vi "Main.vi"() -> ()   [LabVIEW 2018]
uses:
  Controls/1D_2D.ctl
  Controls/Rows_Columns.ctl
  Controls/Lengths_Rows_Columns.ctl
  Controls/E_S.ctl
panel:
  in  "Tab Control":T1(tab)
  in  "Choose Array Size":T2
  in  "Array Size 1D":i8[](array[numeric])=[0, 1, 2, 3]
  in  "Array Size 2D":i8[][](array[numeric])=[[0, 4, 8], [1, 5, 9], [2, 6, 10], [3, 7, 11]]
  out "Size 1D":i32
  out "Size 2D":T3
  in  "Index 1D":i32
  in  "Indexs":T3={"Rows"=-1, "Columns"=-1} {"Columns" min=-1; "Rows" min=-1}
  in  "Index Array 1D":i8[](array[numeric])=[1, 3, 4, -2, 0, 10]
  in  "Index Array 2D":i8[][](array[numeric])=[[0, 4, -3], [1, 5, -4], [2, -1, -5], [3, -2, 100]]
  out "Index Value":i8
  out "Index SubArray":i8[](array[numeric])
  in  "Choose Index Array":T2
  in  "E or S Index Array":T4
  in  "Choose RAS":T2
  in  "Element RAS":i8=-10
  in  "E or S RAS":T4
  in  "Subarray RAS":i8[](array[numeric])=[-5, -8]
  in  "Index RAS":i32
  in  "RAS1D":i8[](array[numeric])=[100, -1, -2, 9, 10]
  in  "RAS2D":i8[][](array[numeric])=[[0, 4, 7], [0, 5, 8], [3, 6, 9]]
  in  "Indexs RAS":T3={"Rows"=-1, "Columns"=-1} {"Columns" min=-1; "Rows" min=-1}
  out "New Array RAS1D":i8[](array[numeric])
  out "New Array RAS2D":i8[][](array[numeric])
  in  "Choose IIA":T2
  in  "E or S IIA":T4
  in  "Index IIA":i32
  in  "Element IIA":i8
  in  "SubArray IIA":i8[](array[numeric])=[-1, -2]
  in  "Insert Into Array 1D":i8[](array[numeric])=[1, 2, 3, 4]
  out "Array 1D IIA":i8[](array[numeric])=[1, 2, 3, 4]
  in  "SubArray IIA 2D":i8[][](array[numeric])=[[-10, -12], [-11, -13]]
  in  "Indexs IIA":T3={"Rows"=-1, "Columns"=-1}
  in  "Insert Into Array 2D":i8[][](array[numeric])=[[0, 3, 6], [1, 4, 7], [2, 5, 8]]
  out "Array 2D IIA":i8[][](array[numeric])
  in  "Choose delete from array":T2
  in  "Length":i32
  in  "Index Delete":i32
  in  "Delete from Array 1D":i8[](array[numeric])=[0, 1, 2, 3, 4]
  in  "Indexs DFA":T3={"Rows"=-1, "Columns"=-1} {"Columns" min=-1; "Rows" min=-1}
  out "New Array 1D":i8[](array[numeric])
  out "Deleted Portion 1D":i8[](array[numeric])
  in  "Delete from Array 2D":i8[][](array[numeric])=[[-5, -1, 3], [-4, 0, 4], [-3, 1, 5], [-2, 2, 6]]
  out "New Array 2D":i8[][](array[numeric])
  out "Deleted Portion 2D":i8[][](array[numeric])
  in  "Choose Initialize Array":T2
  in  "Value":i8
  in  "Dimension 1D Array":i32
  in  "Dimensions for 2D":T3
  out "Initialized Array 1D":i8[](array[numeric])
  out "Initialized Array 2D":i8[][](array[numeric])
  in  "Choose Subset Array":T2
  in  "Index Subset":i32
  in  "Subset Array 1D":i8[](array[numeric])=[0, 1, 2, 3, 4]
  out "SubArray 1D":i8[](array[numeric])
  in  "Length Subset":i32
  in  "Indexs SA":T3={"Rows"=-1, "Columns"=-1} {"Columns" min=-1; "Rows" min=-1}
  in  "Lengths R&C":T5
  in  "Subset Array 2D":i8[][](array[numeric])=[[-5, -1, 3], [-4, 0, 4], [-3, 1, 5], [-2, 2, 6]]
  out "SubArray 2D":i8[][](array[numeric])
  in  "Max & Min Array 1D":i8[](array[numeric])=[1, -1, 2, 100, 10]
  in  "Max & Min Array 2D":i8[][](array[numeric])=[[-3, 55, 41], [6, -1, 14], [-3, 2, -70], [-100, 1, 7]]
  in  "Choose Max & Min Array":T2
  out "Max. Value":i8
  out "Indexs Min.":T3
  out "Index Max.":i32
  out "Indexs Max.":T3
  out "Min. Value":i8
  out "Index Min.":i32
  in  "Sort Array":i8[](array[numeric])=[3, 9, 8, 11, 100, 14]
  out "Sorted Array":i8[](array[numeric])=[3, -7, 8, -3, 100, 14]
  # "Usarán el Tab Control\npara ordenar los controles\ne indicadores necesarios para\ncada sección de la tarea"
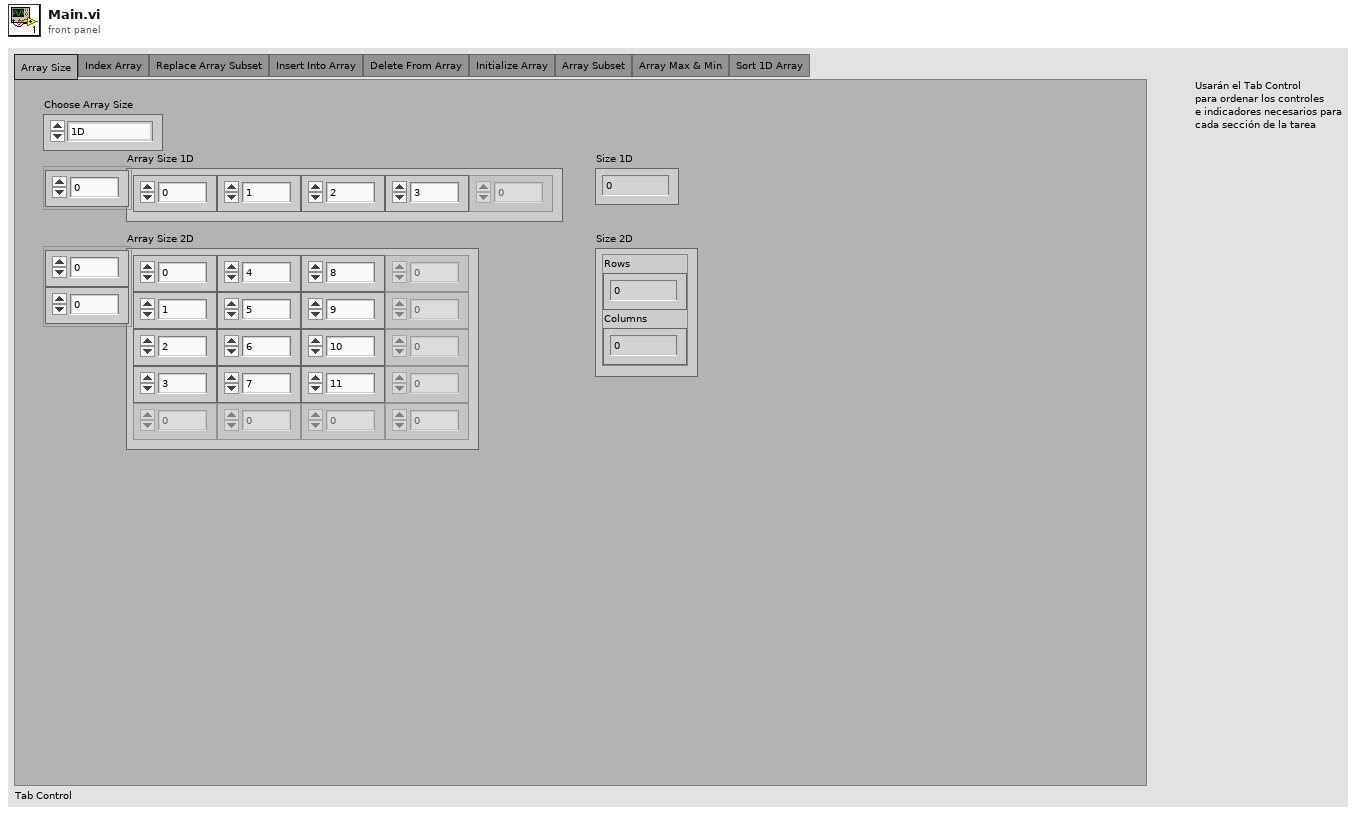
[diagram p1: front panel]
types:
  T1 = enum32{"Array Size", "Index Array", "Replace Array Subset", "Insert Into Array", "Delete From Array", "Initialize Array", "Array Subset", "Array Max & Min", "Sort 1D Array"}
  T2 = typedef "1D_2D.ctl" = enum16{"1D", "2D"}
  T3 = typedef "Rows_Columns.ctl" = cluster{"Rows":i32, "Columns":i32}
  T4 = typedef "E_S.ctl" = enum16{"Element", "SubArray"}
  T5 = typedef "Lengths_Rows_Columns.ctl" = cluster{"Length Rows":i32, "Length Columns":i32}
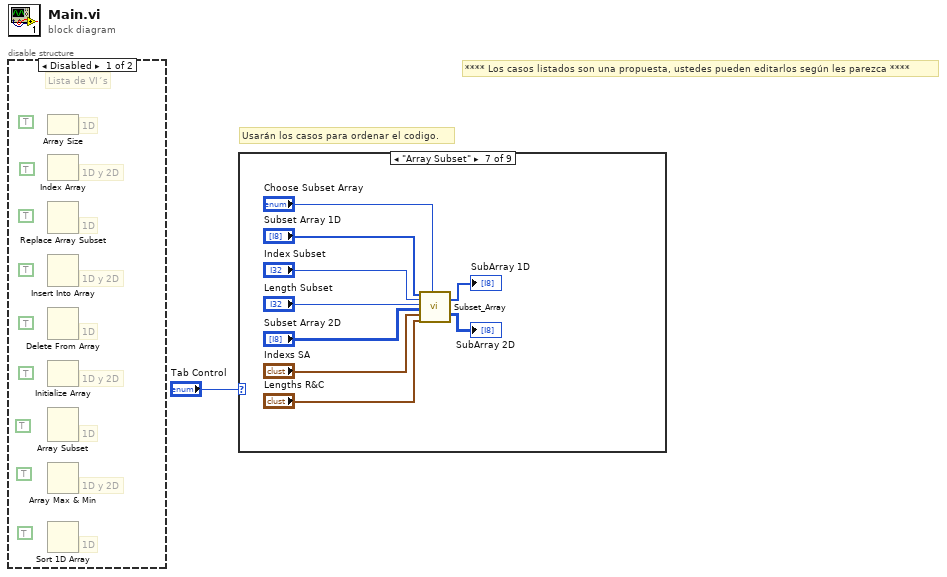
[diagram p0: block diagram]
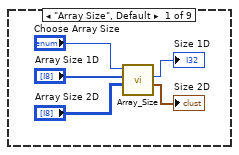
[diagram p3: hidden frame]
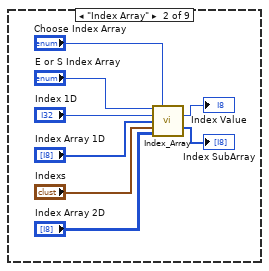
[diagram p4: hidden frame]
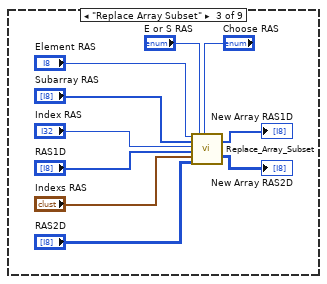
[diagram p5: hidden frame]
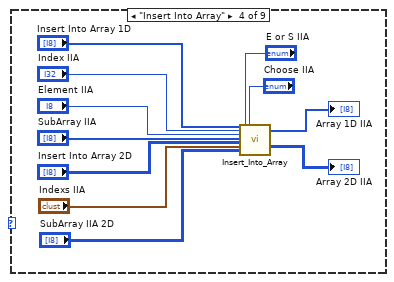
[diagram p6: hidden frame]
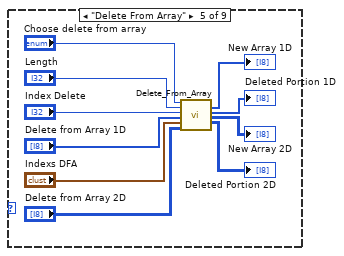
[diagram p7: hidden frame]
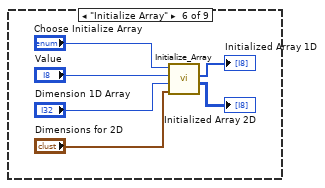
[diagram p8: hidden frame]
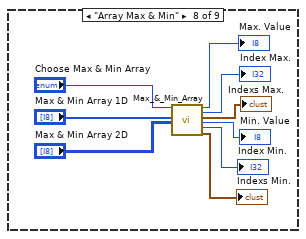
[diagram p9: hidden frame]
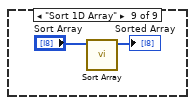
[diagram p10: hidden frame]
diagram:
  # "**** Los casos listados son una propuesta, ustedes pueden editarlos según les parezca ****"
  # "Usarán los casos para ordenar el codigo."
  n1 = disable-structure shown="Disabled" {
    frame Disabled {
      (unwired) TRUE
      (unwired) TRUE
      (unwired) TRUE
      (unwired) TRUE
      (unwired) TRUE
      (unwired) TRUE
      (unwired) TRUE
      (unwired) TRUE
      (unwired) TRUE
      # "Lista de VI´s"
      # "1D"
      # "1D y 2D"
      # "1D"
      # "1D y 2D"
      # "1D"
      # "1D y 2D"
      # "1D"
      # "1D y 2D"
      # "1D"
      n2 = Array Size() -> ()  [unwired: 1 in, 1 out]
      n3 = Index Array "Index Array"() -> ()  [unwired: 2 in, 1 out]
      n4 = Replace Array Subset "Replace Array Subset"() -> ()  [unwired: 3 in, 1 out]
      n5 = Insert Into Array "Insert Into Array"() -> ()  [unwired: 3 in, 1 out]
      n6 = Delete From Array "Delete From Array"() -> ()  [unwired: 3 in, 2 out]
      n7 = Initialize Array "Initialize Array"() -> ()  [unwired: 2 in, 1 out]
      n8 = Array Subset "Array Subset"() -> ()  [unwired: 3 in, 1 out]
      n9 = Array Max & Min() -> ()  [unwired: 1 in, 4 out]
      n10 = Sort 1D Array() -> ()  [unwired: 1 in, 1 out]
    }
    frame Enabled {
    }
  }
  n11 = case shown="\"Array Subset\"" "Tab Control" {
    frame "Array Size", Default {
      n12 = call "Array_Size.vi"("Array Size 2D"="Array Size 2D", "Array Size 1D"="Array Size 1D", "Choose Array Size"="Choose Array Size") -> ("Size 2D"=→"Size 2D":T3, "Size 1D"=→"Size 1D":i32)  [unwired: 7 in]
    }
    frame "Index Array" {
      n13 = call "Index_Array.vi"("E or S Index Array"="E or S Index Array", "Choose Index Array"="Choose Index Array", "Index 1D"="Index 1D", "Index Array 1D"="Index Array 1D", "Indexs Array 2D"="Indexs", "Index Array 2D"="Index Array 2D") -> ("Index Value"=→"Index Value":i8, "Index SubArray"=→"Index SubArray":i8[])  [unwired: 8 in]
    }
    frame "Replace Array Subset" {
      n14 = call "Replace_Array_Subset.vi"("Element RAS"="Element RAS", "Subarray RAS"="Subarray RAS", "Index RAS"="Index RAS", "RAS1D"="RAS1D", "Indexs RAS"="Indexs RAS", "RAS2D"="RAS2D", "E or S RAS"="E or S RAS", "Choose RAS"="Choose RAS") -> ("New Array RAS1D"=→"New Array RAS1D":i8[], "New Array RAS2D"=→"New Array RAS2D":i8[][])  [unwired: 10 in]
    }
    frame "Insert Into Array" {
      n15 = call "Insert_Into_Array.vi"("Insert Into Array 1D"="Insert Into Array 1D", "Index IIA"="Index IIA", "Element IIA"="Element IIA", "SubArray IIA"="SubArray IIA", "Insert Into Array 2D"="Insert Into Array 2D", "Indexs IIA"="Indexs IIA", "SubArray IIA 2D"="SubArray IIA 2D", "E or S IIA"="E or S IIA", "Choose IIA"="Choose IIA") -> ("Array 1D IIA"=→"Array 1D IIA":i8[], "Array 2D IIA"=→"Array 2D IIA":i8[][])  [unwired: 17 in]
    }
    frame "Delete From Array" {
      n16 = call "Delete_From_Array.vi"("Choose delete from array"="Choose delete from array", "Length"="Length", "Index Delete"="Index Delete", "Delete from Array 1D"="Delete from Array 1D", "Indexs DFA"="Indexs DFA", "Delete from Array 2D"="Delete from Array 2D") -> ("New Array 1D"=→"New Array 1D":i8[], "Deleted Portion 1D"=→"Deleted Portion 1D":i8[], "New Array 2D"=→"New Array 2D":i8[][], "Deleted Portion 2D"=→"Deleted Portion 2D":i8[][])  [unwired: 10 in]
    }
    frame "Initialize Array" {
      n17 = call "Initialize_Array.vi"("Dimensions for 2D"="Dimensions for 2D", "Dimension 1D Array"="Dimension 1D Array", "Value"="Value", "Choose Initialize Array"="Choose Initialize Array") -> ("Initialized Array 2D"=→"Initialized Array 2D":i8[][], "Initialized Array 1D"=→"Initialized Array 1D":i8[])  [unwired: 6 in]
    }
    frame "Array Subset" {
      n18 = call "Subset_Array.vi"("Subset Array 1D"="Subset Array 1D", "Index Subset"="Index Subset", "Length Subset"="Length Subset", "Subset Array 2D"="Subset Array 2D", "Indexs SA"="Indexs SA", "Lengths R&C"="Lengths R&C", "Choose Subset Array"="Choose Subset Array") -> ("SubArray 1D"=→"SubArray 1D":i8[], "SubArray 2D"=→"SubArray 2D":i8[][])  [unwired: 11 in]
    }
    frame "Array Max & Min" {
      n19 = call "Max_&_Min_Array.vi"("Choose Max & Min Array"="Choose Max & Min Array", "Max & Min Array 1D"="Max & Min Array 1D", "Max & Min Array 2D"="Max & Min Array 2D") -> ("Max. Value"=→"Max. Value":i8, "Index Max."=→"Index Max.":i32, "Indexs Max."=→"Indexs Max.":T3, "Min. Value"=→"Min. Value":i8, "Index Min."=→"Index Min.":i32, "Indexs Min."=→"Indexs Min.":T3)  [unwired: 11 in]
    }
    frame "Sort 1D Array" {
      n20 = call "Sort Array.vi"("Sort Array"="Sort Array") -> ("Sorted Array"=→"Sorted Array":i8[])  [unwired: 10 in]
    }
  }
